vi "Pre Launch Init.vi"(11 "Nested in":refnum<class "Turnos.lvclass">) -> (0 "error out":errorcluster, 3 "Nested out":refnum<class "Turnos.lvclass">)   [LabVIEW 2020, in "Turnos.lvlib" / "Turnos.lvclass"]
doc: "(<B>Filename</B>: Actor Framework.lvlib:Actor.lvclass:Pre Launch Init.vi)\n\nDefines behavior that occurs after the Launch Nested Actor method is invoked but before the actor's Actor Core method begins running.\n\nBy default, this method does nothing. A descendant class may override it to define behavior."
uses:
  Turnos.lvclass
  C:/Program Files (x86)/National Instruments/LabVIEW 2020/vi.lib/ActorFramework/Actor/Actor.lvclass
  Turnos.lvclass/Turnos.ctl
  <vilib>/ActorFramework/Actor/Actor.lvclass/Actor.ctl
  <vilib>/ActorFramework/Message Enqueuer/Message Enqueuer.lvclass/Message Enqueuer.ctl
  <vilib>/ActorFramework/Message Enqueuer/Init from Existing Queue.vi
  <vilib>/ActorFramework/Message Enqueuer/Enqueue.vi
  Turnos Messages/DRAW FP TURNOS IN UI Msg/DRAW FP TURNOS IN UI Msg.lvclass
  C:/Program Files (x86)/National Instruments/LabVIEW 2020/vi.lib/ActorFramework/Message/Message.lvclass
  <vilib>/ActorFramework/Message Priority Queue/Priority Enqueue.vi
  <vilib>/ActorFramework/Message Enqueuer/Message Enqueuer.lvclass
  <vilib>/ActorFramework/Actor/Actor.lvclass
  Turnos Messages/Delete listbox Msg/Delete listbox Msg.lvclass
  C:/Users/HP/Desktop/Salma_Aguayo/Turnos/Turnos.lvclass
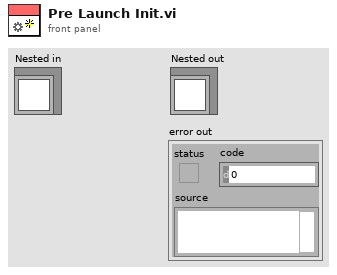
[diagram p1: front panel]
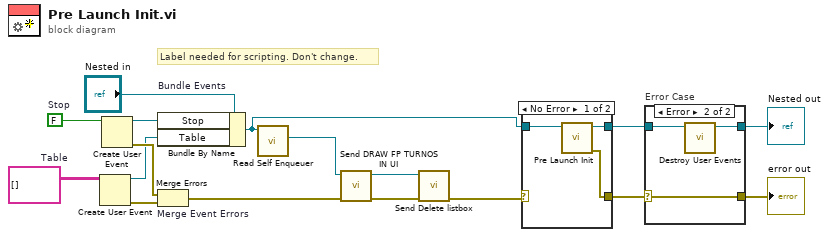
[diagram p0: block diagram]
diagram:
  w6 = string[][] []  # Table
  w16 = FALSE  # Stop
  # "Label needed for scripting. Don't change."
  n1 = Create User Event(user event datatype=w6) -> (user event=w4:refnum<user-event>, error out=w5:errorcluster)  [unwired: 1 in]
  n2 = Create User Event(user event datatype=w16) -> (user event=w13:refnum<user-event>, error out=w15:errorcluster)  [unwired: 1 in]
  n3 = Bundle By Name "Bundle Events"(cluster="Nested in", "Stop"=w13, "Table"=w4) -> (w9:refnum<class "Turnos.lvclass">)
  n4 = Merge Errors "Merge Event Errors"(w15, w5) -> (w7:errorcluster)
  n5 = call <vilib>:"Read Self Enqueuer.vi"("Actor"=w9) -> ("Self Enqueuer"=w8:refnum<class "Message Enqueuer.lvclass">)  [unwired: 10 in]
  n6 = call "Send DRAW FP TURNOS IN UI.vi"("error in (no error)"=w7, "Message Enqueuer"=w8) -> ("error out"=w2:errorcluster, "Message Enqueuer out"=w3:refnum<class "Message Enqueuer.lvclass">)  [unwired: 8 in]
  n7 = call "Send Delete listbox.vi"("error in (no error)"=w2, "Message Enqueuer"=w3) -> ("error out"=w1:errorcluster)  [unwired: 8 in, 1 out]
  n8 = case shown="No Error" w1 {
    selector: w1 -> [_ w22]
    tunnel: [w20 w21] -> w11
    tunnel: w9 -> [w19 w21]
    tunnel: [w18 w22] -> w10
    frame No Error {
      n9 = call-parent "Pre Launch Init.vi"("Actor in"=w19) -> ("error out"=w18:errorcluster, "Actor out"=w20:refnum<class "Turnos.lvclass">)  [unwired: 9 in]
    }
    frame Error {
    }
  }
  n10 = case "Error Case" shown="Error" w10 {
    selector: w10 -> [w23 w27]
    tunnel: w11 -> [w24 w26]
    tunnel: [w24 w25] -> w14
    tunnel: [w23 w27] -> w12
    frame No Error {
    }
    frame Error {
      n11 = call "Destroy User Events.vi"("UI Template in"=w26) -> ("UI Template out"=w25:refnum<class "Turnos.lvclass">)  [unwired: 10 in]
    }
  }
  "error out" <- w12
  "Nested out" <- w14
